vi "Send Serial Command to Camera.vi"(8 "error in (no error)":errorcluster, 10 "String to write":string="str et f", 11 "IMAQ Session In":refnum<k11>) -> (0 "error out":errorcluster, 1 "Confirmation / Error String":string, 2 "Parrot String":string, 3 "IMAQ Session Out":refnum<k11>)   [LabVIEW 2013]
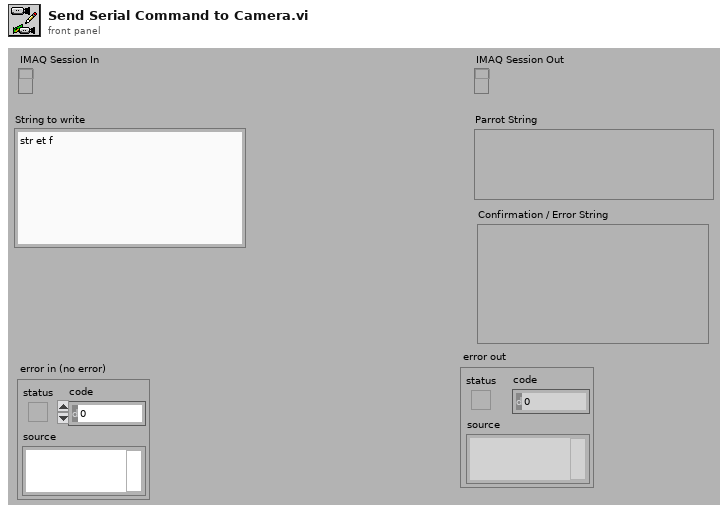
[diagram p1: front panel]
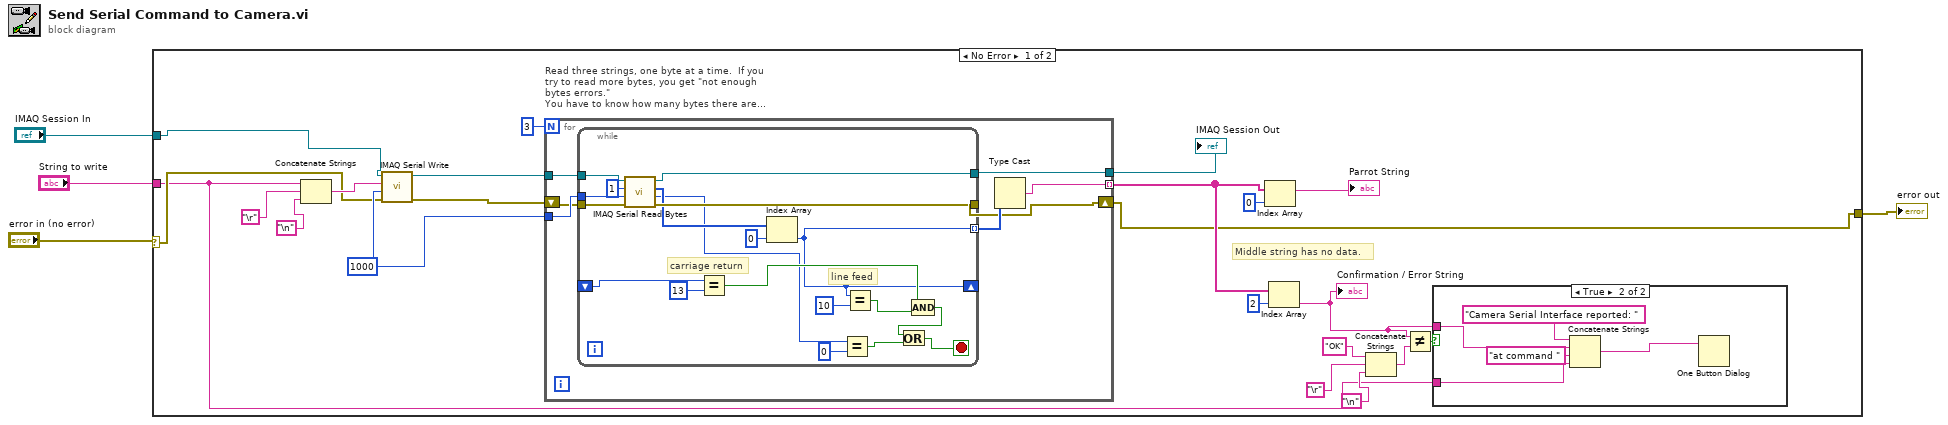
[diagram p0: block diagram]
diagram:
  n1 = case shown="No Error" "error in (no error)" {
    selector: "error in (no error)" -> [w7 w58]
    tunnel: "String to write" -> [w5 _]
    tunnel: "IMAQ Session In" -> [w6 _]
    tunnel: [w14 w58] -> w1
    frame No Error {
      w22 = u32 1000 ("Timeout")
      # "Middle string has no data."
      n2 = Concatenate Strings(w5, "\r", "\n") -> (w26:string)
      n3 = call <vilib>:"IMAQ Serial Write.vi"("error in (no error)"=w7, "Timeout"=w22, "String to write"=w26, "IMAQ Session In"=w6) -> ("error out"=w24:errorcluster, "IMAQ Session Out"=w23:refnum<k11>)  [unwired: 4 in]
      n4 = for "Read three strings, one byte at a time.  If you try to read more bytes, you get \"not enough bytes errors.\"\nYou have to know how many bytes there are before you request them.\nIf you try to use the Imaq Read Serial (that searches for end of line chars from the camera configuration\nfile) the read lines get mangled.  This appears to be a labview bug." {
        N: 3 -> [_]
        tunnel: w23 -> [w38]
        tunnel: w22 -> [w37]
        shift-right: [w34] -> w14
        shift-left: w24 -> [w35]
        tunnel: [w33] -> w15 mode=indexing
        tunnel: [w32] -> w25
        n5 = while {
          tunnel: [w56] -> w32
          tunnel: [w55] -> w34
          tunnel: w38 -> [w54]
          tunnel: w35 -> [w53]
          tunnel: w37 -> [w52]
          shift-right: [w46] -> _
          shift-left: _ -> [w49]
          tunnel: [w46] -> w36 mode=indexing
          stop <- w39 stop-if-true
          # "line feed"
          # "carriage return"
          n6 = call <vilib>:"IMAQ Serial Read Bytes.vi"("error in (no error)"=w53, "Timeout"=w52, "Bytes to Read"=u32 1, "IMAQ Session In"=w54) -> ("error out"=w55:errorcluster, "Bytes Read"=w43:u32, "Byte Array"=w51:i8[], "IMAQ Session Out"=w56:refnum<k11>)  [unwired: 2 in]
          n7 = Equal?(x=w49, y=i8 13) -> (x = y?=w47:bool)
          n8 = Index Array(array=w51, index=0) -> (element=w46:i8)
          n9 = Equal?(x=w43, y=u32 0) -> (x = y?=w41:bool)
          n10 = Equal?(x=w46, y=i8 10) -> (x = y?=w45:bool)
          n11 = Compound Arithmetic op=AND(w47, w45) -> (w40:bool)
          n12 = Or(x=w40, y=w41) -> (x .or. y?=w39:bool)
        }
        n13 = Type Cast(x=w36) -> (*(type *) &x=w33:string)  [unwired: 1 in]
      }
      "IMAQ Session Out" <- w25
      n14 = Index Array(array=w15, index=0) -> (element=→"Parrot String":string)
      n15 = Index Array(array=w15, index=2) -> (element=w11:string)
      "Confirmation / Error String" <- w11
      n16 = Concatenate Strings("OK" ("y"), "\r", "\n") -> (w8:string)
      n17 = Not Equal?(x=w11, y=w8) -> (x != y?=w13:bool)
      n18 = case shown="True" w13 {
        tunnel: w11 -> [_ w30]
        tunnel: w5 -> [_ w27]
        frame False {
        }
        frame True {
          n19 = Concatenate Strings("Camera Serial Interface reported: " ("y"), w30, "at command " ("string"), w27) -> (w29:string)
          n20 = One Button Dialog(message=w29) -> ()  [unwired: 1 in, 1 out]
        }
      }
    }
    frame Error {
    }
  }
  "error out" <- w1
